vi "Queue Actor.vi"(7 "Queue of Self":refnum<queue>, 8 "Self Alias":string, 9 "Caller":refnum<data-value>, 10 "Caller Alias":string, 11 "Queue Actor":refnum<class "Queue Actor.lvclass">) -> ()   [LabVIEW 2021, in "jettl Queue Actor.lvlib" / "jettl Queue Actor.lvclass"]
uses:
  jettl Queue Actor.lvclass
  jettl Queue Actor.lvclass/jettl Queue Actor.ctl
  jettl Queue Actor.lvlib
  Actor/Msgs/Queue Last Ack/Queue Last Ack Msg/Queue Last Ack Msg.lvclass
  Actor/Msgs/Setup/Setup Msg/Setup Msg.lvclass
  Actor/Actor/Actor.lvclass
  C:/git/jettl/src/Actor/Actor/Actor.lvclass
  C:/git/jettl/src/Actor/Msgs/Setup/Setup/Setup.lvclass
  C:/git/jettl/src/Actor/Msgs/Teardown/Teardown/Teardown.lvclass
  C:/git/jettl/src/Actor/Queue Actor/Queue Actor.lvclass
  C:/git/jettl/src/Actor/Msgs/Event Create/Event Create/Event Create.lvclass
  C:/git/jettl/src/Actor/Msgs/Event Last Ack/Event Last Ack/Event Last Ack.lvclass
  C:/git/jettl/src/Actor/Msgs/Queue Create/Queue Create/Queue Create.lvclass
  C:/git/jettl/src/Actor/Msgs/Queue Last Ack/Queue Last Ack/Queue Last Ack.lvclass
  C:/git/jettl/src/jettl/jettl Queue Actor/jettl Queue Actor/jettl Queue Actor.lvclass
  Actor/Msg/Msg.lvclass
  Actor/Queue Actor/Queue Actor.lvclass
  C:/git/jettl/src/Actor/Msgs/Setup/Setup Msg/Setup Msg.lvclass
  C:/git/jettl/src/Actor/Msg/Msg.lvclass
  C:/git/jettl/src/Actor/Msgs/Queue Last Ack/Queue Last Ack Msg/Queue Last Ack Msg.lvclass
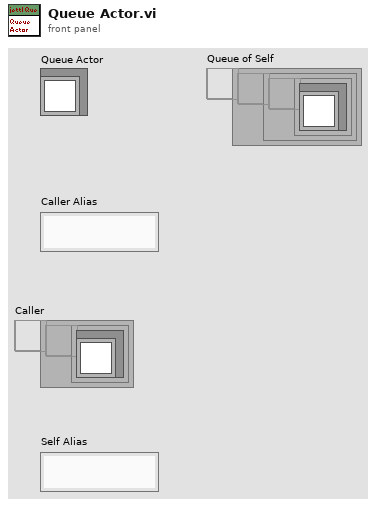
[diagram p1: front panel]
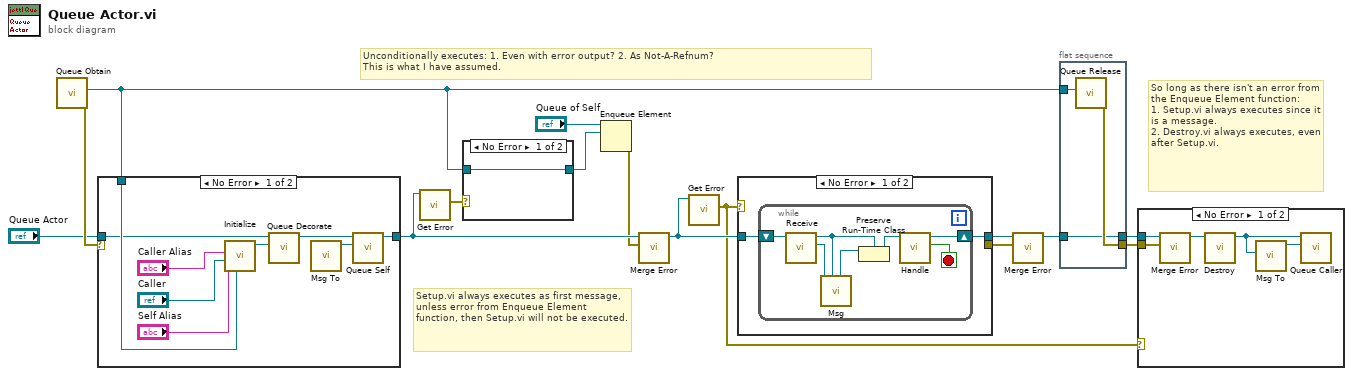
[diagram p0: block diagram]
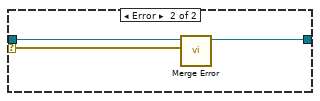
[diagram p4: hidden frame]
diagram:
  # "Unconditionally executes: 1. Even with error output? 2. As Not-A-Refnum?\nThis is what I have assumed."
  # "Setup.vi always executes as first message, unless error from Enqueue Element function, then Setup.vi will not be executed."
  # "So long as there isn't an error from the Enqueue Element function:\n1. Setup.vi always executes since it is a message.\n2. Destroy.vi always executes, even after Setup.vi."
  n1 = call "Queue Obtain.vi"() -> ("error out"=w15:errorcluster, "Queue"=w6:refnum<data-value>)  [unwired: 10 in]
  n2 = case shown="No Error" w15 {
    selector: w15 -> [_ w26]
    tunnel: [w19 w27] -> w5
    tunnel: "Queue Actor" -> [w18 w25]
    tunnel: w6 -> [w24 _]
    frame No Error {
      n3 = call "Initialize.vi"("Self"=w24, "Self Alias"="Self Alias", "Caller"="Caller", "Caller Alias"="Caller Alias") -> ("jettl Queue Actor out"=w16:refnum<class "jettl Queue Actor.lvclass">)  [unwired: 7 in]
      n4 = call-dynamic "Queue Decorate.vi"("Queue Actor"=w16, "Queue Actor in"=w18) -> ("Queue Actor out"=w17:refnum<class "Queue Actor.lvclass">)  [unwired: 9 in]
      n5 = call "Msg To.vi"() -> ("Setup Msg out"=w20:refnum<class "Setup Msg.lvclass">)  [unwired: 11 in]
      n6 = call-dynamic "Queue Self.vi"("Msg"=w20, "Actor in"=w17) -> ("Actor out"=w19:refnum<class "Queue Actor.lvclass">)  [unwired: 9 in]
    }
    frame Error {
      n7 = call-dynamic "Merge Error.vi"("Error"=w26, "Set Error in"=w25) -> ("Set Error out"=w27:refnum<class "Queue Actor.lvclass">)  [unwired: 9 in]
    }
  }
  n8 = call-dynamic "Get Error.vi"("Actor in"=w5) -> ("Error"=w8:errorcluster)  [unwired: 10 in]
  n9 = case shown="No Error" w8 {
    tunnel: [w28 _] -> w7
    tunnel: w6 -> [w28 _]
    frame No Error {
    }
    frame Error {
    }
  }
  n10 = Enqueue Element(queue="Queue of Self", element=w7) -> (error out=w3:errorcluster)  [unwired: 2 in, 2 out]
  n11 = call-dynamic "Merge Error.vi"("Error"=w3, "Set Error in"=w5) -> ("Set Error out"=w4:refnum<class "Queue Actor.lvclass">)  [unwired: 9 in]
  n12 = call-dynamic "Get Error.vi"("Actor in"=w4) -> ("Error"=w2:errorcluster)  [unwired: 10 in]
  n13 = case shown="No Error" w2 {
    selector: w2 -> [_ w39]
    tunnel: w4 -> [w30 w38]
    tunnel: [w29 w38] -> w14
    tunnel: [_ w39] -> w12
    frame No Error {
      n14 = while {
        shift-right: [w37] -> w29
        shift-left: w30 -> [w35]
        stop <- w36 stop-if-true
        n15 = call-dynamic "Receive.vi"("Actor in"=w35) -> ("Msg"=w34:refnum<class "Msg.lvclass">, "Actor out"=w32:refnum<class "Actor.lvclass">)  [unwired: 9 in]
        n16 = call-dynamic "Msg.vi"("Actor in"=w32, "Msg in"=w34) -> ("Actor out"=w33:refnum<class "Actor.lvclass">)  [unwired: 9 in]
        n17 = Preserve Run-Time Class(object in=w33, 2:w32) -> (object out=w31:refnum<class "Actor.lvclass">)  [unwired: 1 in, 1 out]
        n18 = call-dynamic "Handle.vi"("Actor in"=w31) -> ("Destroy?"=w36:bool, "Actor out"=w37:refnum<class "Actor.lvclass">)  [unwired: 9 in]
      }
    }
    frame Error {
    }
  }
  n19 = call-dynamic "Merge Error.vi"("Error"=w12, "Set Error in"=w14) -> ("Set Error out"=w13:refnum<class "Actor.lvclass">)  [unwired: 9 in]
  n20 = flat-sequence {
    tunnel: w6 -> [w42]
    tunnel: [w41] -> w11
    tunnel: [w40] -> w10
    tunnel: w13 -> [w40]
    frame #0 {
      n21 = call "Queue Release.vi"("Queue"=w42) -> ("error out"=w41:errorcluster)  [unwired: 10 in]
    }
  }
  n22 = case shown="No Error" w2 {
    tunnel: w10 -> [w45 _]
    tunnel: w11 -> [w46 _]
    frame No Error {
      n23 = call-dynamic "Merge Error.vi"("Error"=w46, "Set Error in"=w45) -> ("Set Error out"=w43:refnum<class "Actor.lvclass">)  [unwired: 9 in]
      n24 = call-dynamic "Destroy.vi"("Actor in"=w43) -> ("Actor out"=w44:refnum<class "Actor.lvclass">)  [unwired: 10 in]
      n25 = call "Msg To.vi"("Queue Actor"=w44) -> ("Queue Last Ack Msg out"=w47:refnum<class "Queue Last Ack Msg.lvclass">)  [unwired: 10 in]
      n26 = call-dynamic "Queue Caller.vi"("Msg"=w47, "Actor in"=w44) -> ()  [unwired: 9 in, 1 out]
    }
    frame Error {
    }
  }
